vi "CRYOption Setting.vi"() -> (1 "Language Mode Change":bool, 2 "Launch Mode Change":bool, 3 "OK Flag":bool)   [LabVIEW 2013]
uses:
  CRYMainGlobal.vi
  CRYSystem/Acquisition/SubVI/CRYAcquisition Global.vi
  CRYSystem/Program/CRYRef nums global.vi
  Kernel32.DLL
panel:
  in  "Cancel":bool
  in  "OK":bool
  in  "Configure Tab":enum32{"General", "Path Information"}(tab)
  in  "Test Mode":bool
  out "Language Selection":bool caption="语言选择"
  in  "Language Mode":u16(slide) caption="File Name Mode1"
  in  "Language":u16(ring) caption="窗口模式选择" items=["English", "Chinese"]
  in  "Skin Mode Selection":u16(ring) caption="窗口模式选择" items=["Back Mode", "White Mode", "Smart Mode", "General Mode"]
  in  "Demo Mode":bool caption="演示模式"
  in  "CRYoundLab Switch":enum32{"CRY6181", "CRY6181 One"}(radio) caption="GVSoundLab Switch"
  in  "Default Button":bool
  out "SoundCard Path":path caption="硬件路径"
  out "System Path":path caption="系统路径"
  in  "Task Sequence Path":path caption="任务序列路径"
  out "Steps Path":path caption="步骤路径"
  out "Calibration Path":path caption="校准路径"
  in  "Results Path":path caption="结果路径"
  out "Display Path":path caption="显示路径"
  in  "Data Path":path caption="数据路径"
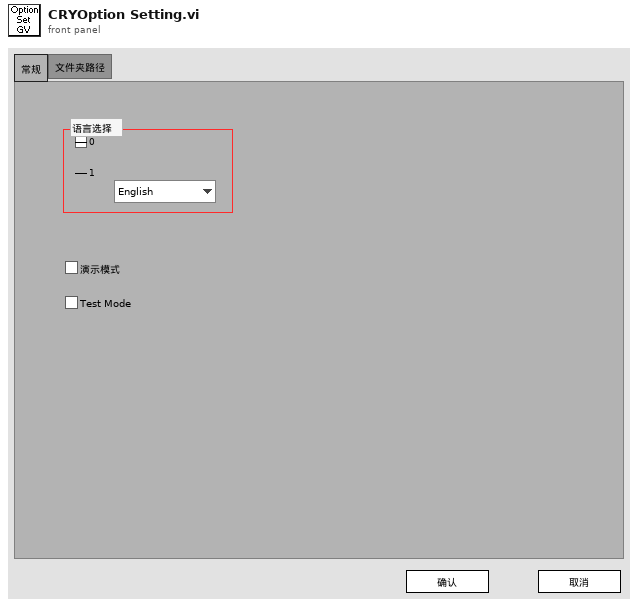
[diagram p1: front panel]
types:
  T1 = cluster{"Section":string, "Item":cluster{"Key":string, "Value":string}[]}
  T2 = enum32{"English", "Chinese", "Korean", "Japanese", "Russian", "Chinese traditional"}
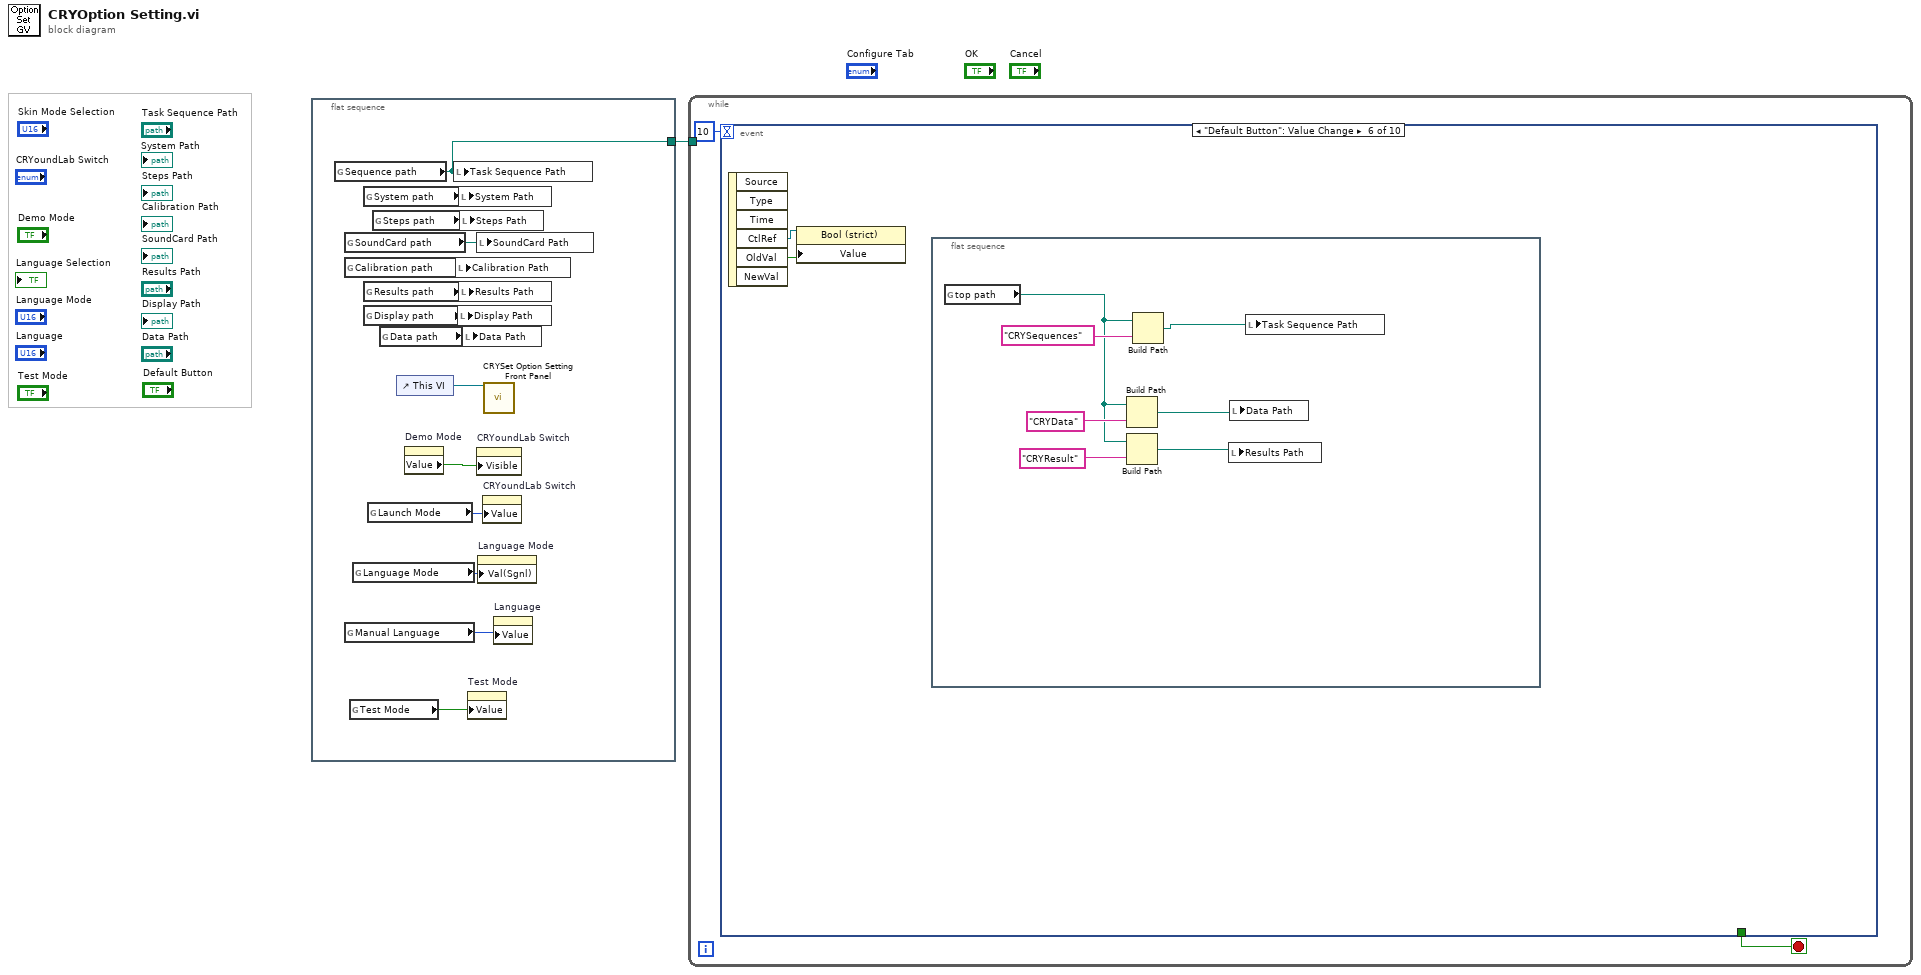
[diagram p0: block diagram]
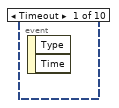
[diagram p2: hidden frame]
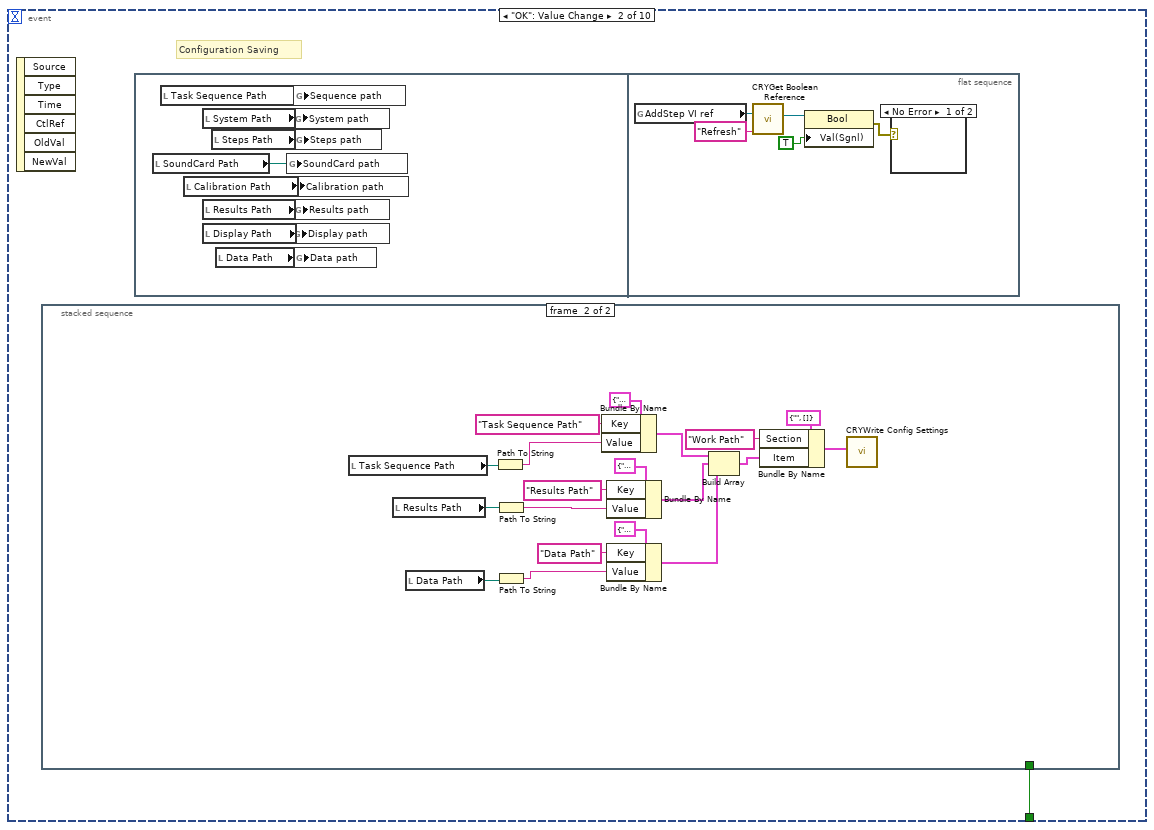
[diagram p3: hidden frame]
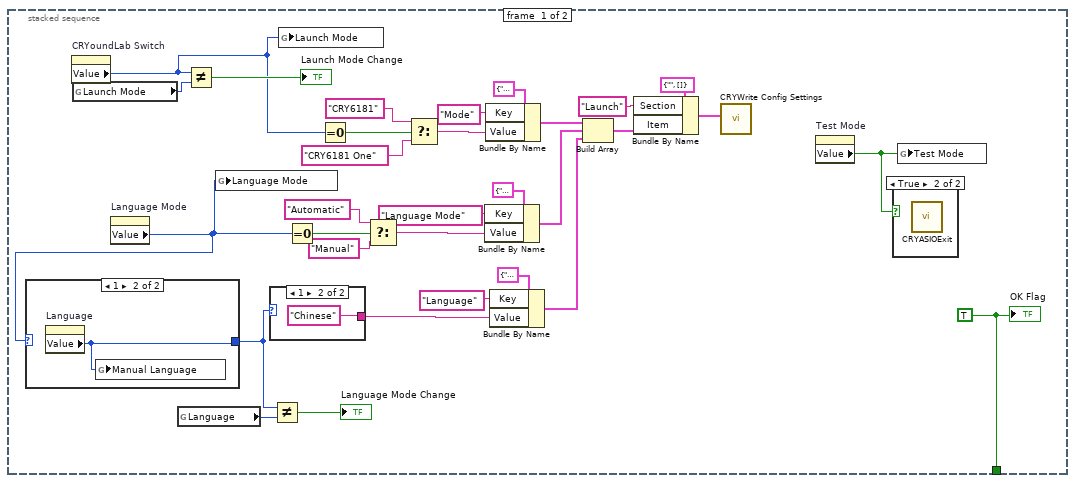
[diagram p4: hidden frame]
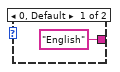
[diagram p6: hidden frame]
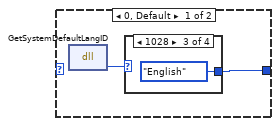
[diagram p7: hidden frame]
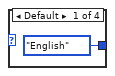
[diagram p8: hidden frame]
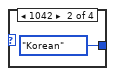
[diagram p9: hidden frame]
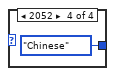
[diagram p10: hidden frame]
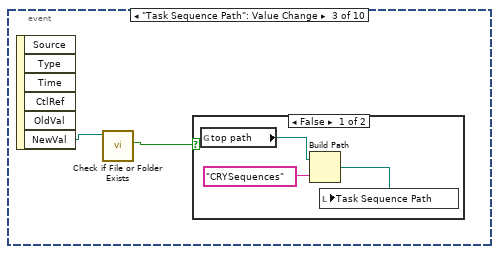
[diagram p12: hidden frame]
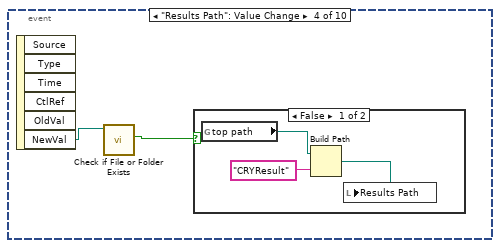
[diagram p14: hidden frame]
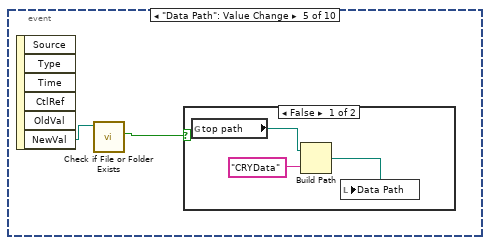
[diagram p16: hidden frame]
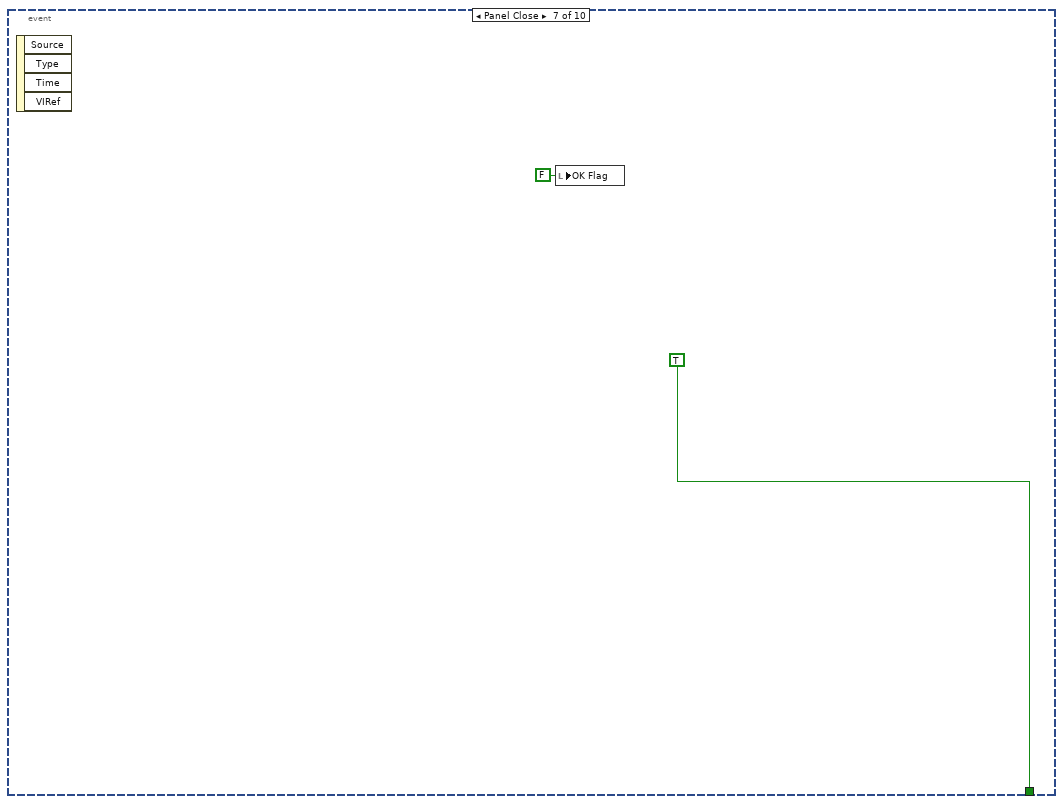
[diagram p18: hidden frame]
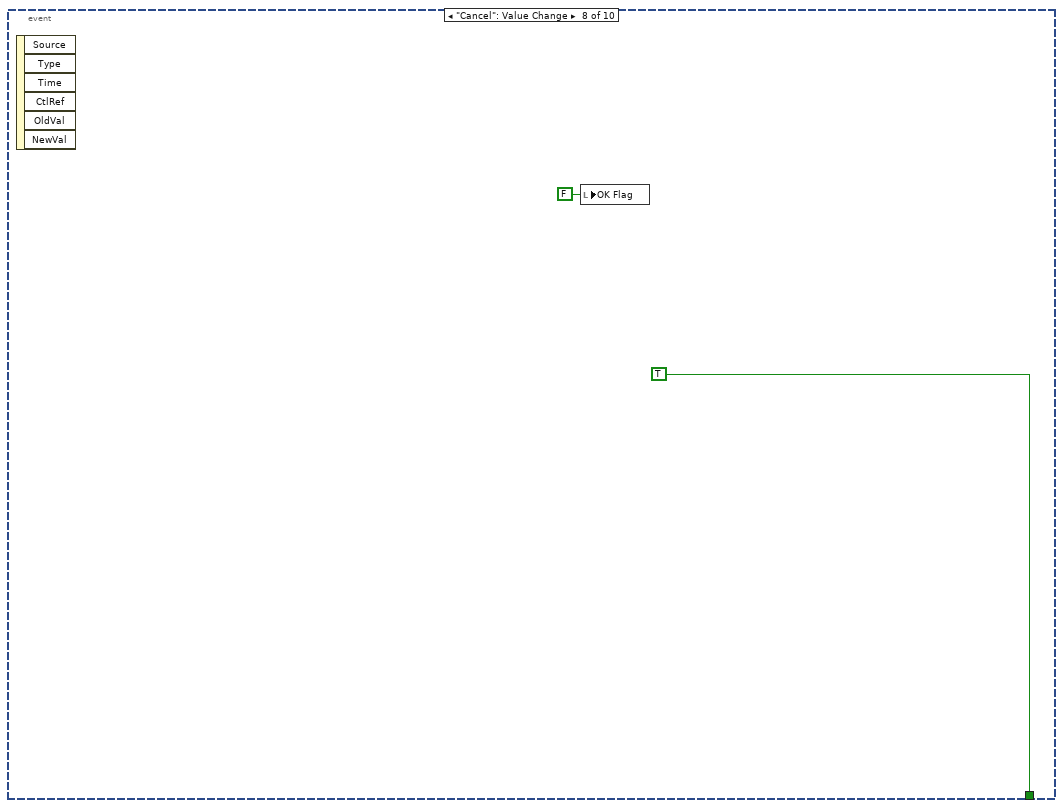
[diagram p19: hidden frame]
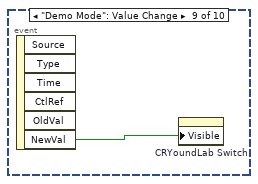
[diagram p20: hidden frame]
diagram:
  n1 = flat-sequence {
    tunnel: [w8] -> w1
    frame #0 {
      n2 = global read "CRYMainGlobal.vi" "Sequence path"() -> (w8:path)
      n3 = global read "CRYMainGlobal.vi" "SoundCard path"() -> (w15:path)
      n4 = global read "CRYMainGlobal.vi" "Calibration path"() -> (w13:path)
      n5 = global read "CRYMainGlobal.vi" "Manual Language"() -> (w3:enum32{"English", "Chinese"})
      n6 = global read "CRYAcquisition Global.vi" "Test Mode"() -> (w2:bool)
      n7 = global read "CRYMainGlobal.vi" "Language Mode"() -> (w4:enum32{"Automatic", "Manual"})
      n8 = global read "CRYMainGlobal.vi" "System path"() -> (w9:path)
      n9 = global read "CRYMainGlobal.vi" "Results path"() -> (w12:path)
      n10 = global read "CRYMainGlobal.vi" "Display path"() -> (w11:path)
      n11 = global read "CRYMainGlobal.vi" "Launch Mode"() -> (w5:enum32{"CRY6181", "CRY6181 One"})
      n12 = global read "CRYMainGlobal.vi" "Steps path"() -> (w10:path)
      n13 = global read "CRYMainGlobal.vi" "Data path"() -> (w14:path)
      n14 = control-ref of="This VI"() -> (w7:refnum<vi>)
      n15 = property on="Demo Mode" class="Bool (strict)"() -> ("Value"=w6:bool)  [unwired: 2 in, 2 out]
      n16 = local write "Task Sequence Path"(w8) -> ()
      n17 = local write "Calibration Path"(w13) -> ()
      n18 = local write "Display Path"(w11) -> ()
      n19 = local write "System Path"(w9) -> ()
      n20 = local write "Results Path"(w12) -> ()
      n21 = local write "Steps Path"(w10) -> ()
      n22 = local write "Data Path"(w14) -> ()
      n23 = property on="Test Mode" class="Bool (strict)"("Value"=w2) -> ()  [unwired: 2 in, 2 out]
      n24 = local write "SoundCard Path"(w15) -> ()
      n25 = property on="CRYoundLab Switch" class="RadioBtnsControl (strict)"("Visible"=w6) -> ()  [unwired: 2 in, 2 out]
      n26 = property on="Language Mode" class="Slide (strict)"("Val(Sgnl)"=w4) -> ()  [unwired: 2 in, 2 out]
      n27 = property on="CRYoundLab Switch" class="RadioBtnsControl (strict)"("Value"=w5) -> ()  [unwired: 2 in, 2 out]
      n28 = call "CRYSet Option Setting Front Panel.vi"("Vi Ref in"=w7) -> ()  [unwired: 10 in, 1 out]
      n29 = property on="Language" class="Ring (strict)"("Value"=w3) -> ()  [unwired: 2 in, 2 out]
    }
  }
  n30 = while {
    tunnel: w1 -> [_]
    stop <- w17 stop-if-true
    n31 = event shown="[5] \"Default Button\": Value Change" {
      selector: _ -> [_ _ _ _ _ _ _ _ _ _]
      dyn-events: _ -> [_ _ _ _ _ _ _ _ _ _]
      timeout: 10 -> [_ _ _ _ _ _ _ _ _ _]
      tunnel: [_ w18 _ _ _ _ TRUE TRUE _ _] -> w17
      event Timeout {
        n32 = event-data() -> ()  [unwired: 3 out]
      }
      event "OK": Value Change {
        # "Configuration Saving"
        n33 = event-data() -> ()  [unwired: 7 out]
        n34 = stacked-sequence {
          tunnel: [w49 _] -> w18
          frame #0 {
            w49 = TRUE
            n35 = property on="CRYoundLab Switch" class="RadioBtnsControl (strict)"() -> ("Value"=w47:enum32{"CRY6181", "CRY6181 One"})  [unwired: 2 in, 2 out]
            n36 = global read "CRYMainGlobal.vi" "Launch Mode"() -> (w29:enum32{"CRY6181", "CRY6181 One"})
            n37 = property on="Language Mode" class="Slide (strict)"() -> ("Value"=w24:u16)  [unwired: 2 in, 2 out]
            n38 = case shown="1" w24 {
              tunnel: [w52 w58] -> w22
              frame 0, Default {
                n39 = dll-call lib="kernel32.dll" fn="GetSystemDefaultLangID"() -> ("return type"=w53:u16)  [unwired: 3 in, 2 out]
                n40 = case shown="1028" w53 {
                  tunnel: [T2."English" ("Language") T2."Korean" ("Language") T2."English" ("Language") T2."Chinese" ("Language")] -> w52
                  frame Default {
                  }
                  frame 1042 {
                  }
                  frame 1028 {
                  }
                  frame 2052 {
                  }
                }
              }
              frame 1 {
                n41 = property on="Language" class="Ring (strict)"() -> ("Value"=w58:u16)  [unwired: 2 in, 2 out]
                n42 = global write "CRYMainGlobal.vi" "Manual Language"(w58) -> ()
              }
            }
            n43 = global read "CRYMainGlobal.vi" "Language"() -> (w23:T2)
            n44 = Not Equal?(x=w47, y=w29) -> (x != y?=→"Launch Mode Change":bool)
            n45 = global write "CRYMainGlobal.vi" "Language Mode"(w24) -> ()
            n46 = case shown="1" w22 {
              tunnel: ["English" ("Section") "Chinese" ("Section")] -> w21
              frame 0, Default {
              }
              frame 1 {
              }
            }
            n47 = Not Equal?(x=w22, y=w23) -> (x != y?=→"Language Mode Change":bool)
            n48 = global write "CRYMainGlobal.vi" "Launch Mode"(w47) -> ()
            n49 = Equal To 0?(x=w24) -> (x = 0?=w44:bool)
            n50 = Equal To 0?(x=w47) -> (x = 0?=w34:bool)
            n51 = Select(t="Automatic" ("Section"), s=w44, f="Manual" ("Section")) -> (s? t:f=w43:string)
            n52 = Select(t="CRY6181" ("Section"), s=w34, f="CRY6181 One" ("Section")) -> (s? t:f=w33:string)
            n53 = Bundle By Name(cluster=cluster{"Key":string, "Value":string} {"Key"="", "Value"=""} ("Cluster"), "Key"="Language Mode" ("Section"), "Value"=w43) -> (w28:cluster{"Key":string, "Value":string})
            n54 = Bundle By Name(cluster=cluster{"Key":string, "Value":string} {"Key"="", "Value"=""} ("Cluster"), "Key"="Mode" ("Section"), "Value"=w33) -> (w38:cluster{"Key":string, "Value":string})
            n55 = Bundle By Name(cluster=cluster{"Key":string, "Value":string} {"Key"="", "Value"=""} ("Cluster"), "Key"="Language" ("Section"), "Value"=w21) -> (w25:cluster{"Key":string, "Value":string})
            n56 = Build Array(w38, w28, w25) -> (w37:cluster{"Key":string, "Value":string}[])
            n57 = Bundle By Name(cluster=T1 {"Section"="", "Item"=[]}, "Section"="Launch", "Item"=w37) -> (w30:T1)
            n58 = call "CRYWrite Config Settings.vi"("Config Data"=w30) -> ()  [unwired: 8 in, 1 out]
            n59 = property on="Test Mode" class="Bool (strict)"() -> ("Value"=w19:bool)  [unwired: 2 in, 2 out]
            n60 = case shown="True" w19 {
              frame False {
              }
              frame True {
                n61 = call "CRYASIOExit.vi"() -> ()  [unwired: 10 in, 2 out]
              }
            }
            n62 = global write "CRYAcquisition Global.vi" "Test Mode"(w19) -> ()
            "OK Flag" <- w49
          }
          frame #1 {
            n63 = local read "Task Sequence Path"() -> (w74:path)
            n64 = local read "Results Path"() -> (w73:path)
            n65 = local read "Data Path"() -> (w72:path)
            n66 = Path To String(path=w74) -> (string=w68:string)
            n67 = Path To String(path=w73) -> (string=w65:string)
            n68 = Path To String(path=w72) -> (string=w62:string)
            n69 = Bundle By Name(cluster=cluster{"Key":string, "Value":string} {"Key"="", "Value"=""} ("Cluster"), "Key"="Task Sequence Path", "Value"=w68) -> (w61:cluster{"Key":string, "Value":string})
            n70 = Bundle By Name(cluster=cluster{"Key":string, "Value":string} {"Key"="", "Value"=""} ("Cluster"), "Key"="Results Path", "Value"=w65) -> (w60:cluster{"Key":string, "Value":string})
            n71 = Bundle By Name(cluster=cluster{"Key":string, "Value":string} {"Key"="", "Value"=""} ("Cluster"), "Key"="Data Path", "Value"=w62) -> (w59:cluster{"Key":string, "Value":string})
            n72 = Build Array(w61, w60, w59) -> (w71:cluster{"Key":string, "Value":string}[])
            n73 = Bundle By Name(cluster=T1 {"Section"="", "Item"=[]}, "Section"="Work Path", "Item"=w71) -> (w75:T1)
            n74 = call "CRYWrite Config Settings.vi"("Config Data"=w75) -> ()  [unwired: 8 in, 1 out]
          }
        }
        n75 = flat-sequence {
          frame #0 {
            n76 = local read "SoundCard Path"() -> (w78:path)
            n77 = local read "Task Sequence Path"() -> (w79:path)
            n78 = local read "Calibration Path"() -> (w85:path)
            n79 = local read "System Path"() -> (w80:path)
            n80 = local read "Results Path"() -> (w84:path)
            n81 = local read "Display Path"() -> (w83:path)
            n82 = local read "Steps Path"() -> (w81:path)
            n83 = local read "Data Path"() -> (w82:path)
            n84 = global write "CRYMainGlobal.vi" "SoundCard path"(w78) -> ()
            n85 = global write "CRYMainGlobal.vi" "Calibration path"(w85) -> ()
            n86 = global write "CRYMainGlobal.vi" "Display path"(w83) -> ()
            n87 = global write "CRYMainGlobal.vi" "System path"(w80) -> ()
            n88 = global write "CRYMainGlobal.vi" "Results path"(w84) -> ()
            n89 = global write "CRYMainGlobal.vi" "Sequence path"(w79) -> ()
            n90 = global write "CRYMainGlobal.vi" "Steps path"(w81) -> ()
            n91 = global write "CRYMainGlobal.vi" "Data path"(w82) -> ()
          }
          frame #1 {
            n92 = global read "CRYRef nums global.vi" "AddStep VI ref"() -> (w90:refnum<vi>)
            n93 = call "CRYGet Boolean Reference.vi"("Label Name"="Refresh", "VI Refnum"=w90) -> ("Boolean Ref"=w88:refnum<vi>)  [unwired: 7 in, 2 out]
            n94 = property class="Bool"(reference=w88, "Val(Sgnl)"=TRUE) -> (error out=w86:errorcluster)  [unwired: 1 in, 1 out]
            n95 = case shown="No Error" w86 {
              frame No Error {
              }
              frame Error {
              }
            }
          }
        }
      }
      event "Task Sequence Path": Value Change {
        n96 = event-data() -> ("NewVal"=w92:path)  [unwired: 6 out]
        n97 = call <vilib>:"Check if File or Folder Exists.vi"("path"=w92) -> ("file or folder exists?"=w91:bool)  [unwired: 8 in, 2 out]
        n98 = case shown="False" w91 {
          frame False {
            n99 = global read "CRYMainGlobal.vi" "top path"() -> (w94:path)
            n100 = Build Path(base path=w94, name or relative path="CRYSequences") -> (appended path=w93:path)
            n101 = local write "Task Sequence Path"(w93) -> ()
          }
          frame True {
          }
        }
      }
      event "Results Path": Value Change {
        n102 = event-data() -> ("NewVal"=w96:path)  [unwired: 6 out]
        n103 = call <vilib>:"Check if File or Folder Exists.vi"("path"=w96) -> ("file or folder exists?"=w97:bool)  [unwired: 8 in, 2 out]
        n104 = case shown="False" w97 {
          frame False {
            n105 = global read "CRYMainGlobal.vi" "top path"() -> (w99:path)
            n106 = Build Path(base path=w99, name or relative path="CRYResult") -> (appended path=w98:path)
            n107 = local write "Results Path"(w98) -> ()
          }
          frame True {
          }
        }
      }
      event "Data Path": Value Change {
        n108 = event-data() -> ("NewVal"=w101:path)  [unwired: 6 out]
        n109 = call <vilib>:"Check if File or Folder Exists.vi"("path"=w101) -> ("file or folder exists?"=w102:bool)  [unwired: 8 in, 2 out]
        n110 = case shown="False" w102 {
          frame False {
            n111 = global read "CRYMainGlobal.vi" "top path"() -> (w104:path)
            n112 = Build Path(base path=w104, name or relative path="CRYData") -> (appended path=w103:path)
            n113 = local write "Data Path"(w103) -> ()
          }
          frame True {
          }
        }
      }
      event "Default Button": Value Change {
        n114 = event-data() -> ("CtlRef"=w107:refnum<vi>, "OldVal"=w106:bool)  [unwired: 5 out]
        n115 = property class="Bool (strict)"(reference=w107, "Value"=w106) -> ()  [unwired: 1 in, 2 out]
        n116 = flat-sequence {
          frame #0 {
            n117 = global read "CRYMainGlobal.vi" "top path"() -> (w110:path)
            n118 = Build Path(base path=w110, name or relative path="CRYData") -> (appended path=w108:path)
            n119 = Build Path(base path=w110, name or relative path="CRYResult") -> (appended path=w109:path)
            n120 = Build Path(base path=w110, name or relative path="CRYSequences") -> (appended path=w111:path)
            n121 = local write "Results Path"(w109) -> ()
            n122 = local write "Data Path"(w108) -> ()
            n123 = local write "Task Sequence Path"(w111) -> ()
          }
        }
      }
      event Panel Close {
        n124 = event-data() -> ()  [unwired: 5 out]
        n125 = local write "OK Flag"(FALSE ("Boolean")) -> ()
      }
      event "Cancel": Value Change {
        n126 = event-data() -> ()  [unwired: 7 out]
        n127 = local write "OK Flag"(FALSE ("Boolean")) -> ()
      }
      event "Demo Mode": Value Change {
        n128 = event-data() -> ("NewVal"=w119:bool)  [unwired: 6 out]
        n129 = property on="CRYoundLab Switch" class="RadioBtnsControl (strict)"("Visible"=w119) -> ()  [unwired: 2 in, 2 out]
      }
      event "Language Mode": Value Change {
        n130 = event-data() -> ("NewVal"=w121:u16)  [unwired: 6 out]
        n131 = case shown="0, Default" w121 {
          tunnel: [FALSE TRUE] -> w120
          frame 0, Default {
          }
          frame 1 {
          }
        }
        n132 = property on="Language" class="Ring (strict)"("Visible"=w120) -> ()  [unwired: 2 in, 2 out]
      }
    }
  }
